vi "RT_test_ADC.vi"() -> ()   [LabVIEW 2018]
uses:
  <vilib>/Platform/TimedLoop/XDataNode/timing_clust.ctl
  <vilib>/Platform/TimedLoop/XDataNode/nitl_modes.ctl
  <vilib>/Platform/TimedLoop/XDataNode/wakeup.ctl
  Type Defs/BL Measurement States.ctl
  <vilib>/FPGAPlugInAG/myRIO-1900/niLvFpga_Open_myRIO-1900.vi
  <vilib>/rvi/interface/common/dynamic/niFpgaDynamicAddResources.vi
  <vilib>/Utility/error.llb/Error Cluster From Error Code.vi
  <vilib>/rvi/errors/niLvFpgaAdjustHostInterfaceError.vi
  <vilib>/rvi/interface/nirviOpenFPGA/nirviOpenFPGA.xnode
  UNCC Watt balance Oct19/FPGA Bitfiles/UNCCWattbalanceO_FPGATarget_fpganestedFORW&R_sb-Oe1PDHtY.lvbitx
  <vilib>/Platform/TimedLoop/XDataNode/XDataNode.xnode
  <vilib>/rvi/interface/nirviReadWriteControl/nirviReadWriteControl.xnode
  <vilib>/Platform/TimedLoop/XDataNode/XDNodeRunTimeDep.lvlib
  NiFpgaLv.dll
  <vilib>/rvi/interface/Simulation/niFpgaSimulationCallBeginRW.vi
panel:
  out "number of cycles":dbl
  out "Time period":dbl
  in  "no. datapoints":u16=1
  in  "gain":dbl=5.7903
  out "Velocity (m/s) 2":dbl=0.0007038140090386572
  out "displacement amplitude":dbl=0.0001120154785558262 format="%.6f"
  out "d input to Fourier":dbl[](graph)
  in  "Measure 2":bool
  out "Waveform Chart - Dark 2":dbl(graph)=-1.5424874498374959 caption="Waveform Chart - dark"
  out "Waveform Chart - Dark":dbl(graph)=0.00010993789767612186 caption="Waveform Chart - dark"
  out "Late? [i-1]":bool
  in  "delay (us)":u32=250
  in  "offset (mV)":dbl
  in  "amplitude (V)":dbl=0.8
  in  "frequency (Hz)":dbl=25.0
  in  "Stop Button":bool
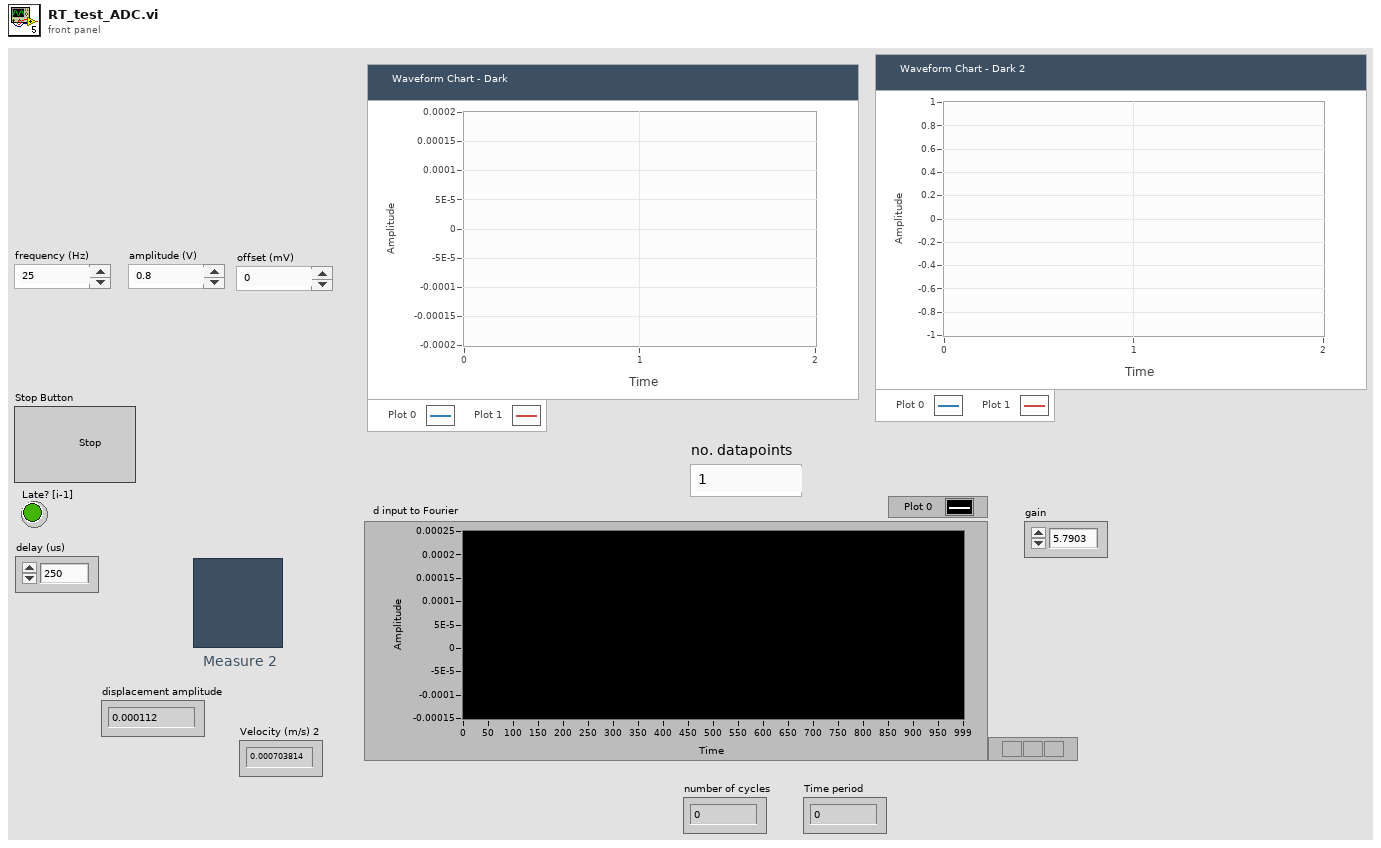
[diagram p1: front panel]
types:
  T1 = typedef "XDNodeRunTimeDep.lvlib/timing_clust.ctl" = cluster{"Expected End [f-1]":u64, "Actual End [f-1]":u64, "Finished Late? [f-1]":bool, "Expected End [i-1]":u64, "Actual End [i-1]":u64, "Finished Late? [i-1]":bool, "Expected Start [i]":u64, "Actual Start [i]":u64, "Expected Start [f]":u64, "Actual Start [f]":u64, "Source Name":string, "Structure Name":string, "Period":i64, "Deadline":i64, "Offset":i64, "Start":i64, "Priority":i32, "Timeout":i32, "Mode":T2, "Wakeup Reason":T3, "Error":errorcluster, "Source Type":string, "Secondary Source Type":string, "Global End Time":u64, "Global Start Time":u64, "Frame Duration":u64, "Iteration Duration":u64, "Assigned CPU":i32, "I/O Scan Engine Mode":u32}
  T2 = typedef "XDNodeRunTimeDep.lvlib/nitl_modes.ctl" = enum32{"No Change", "Process missed periods, maintain original phase", "Discard missed periods, maintain original phase", "Process missed periods, ignore original phase", "Discard missed periods, ignore original phase"}
  T3 = typedef "XDNodeRunTimeDep.lvlib/wakeup.ctl" = enum32{"Normal", "Aborted", "Asynchronous wakeup", "Timing source error", "Timed loop error", "Timeout"}
  T4 = typedef "BL Measurement States.ctl" = enum16{"idle", "initialize", "collect data", "prepare data", "fit sine", "calculate BL", "exit meas"}
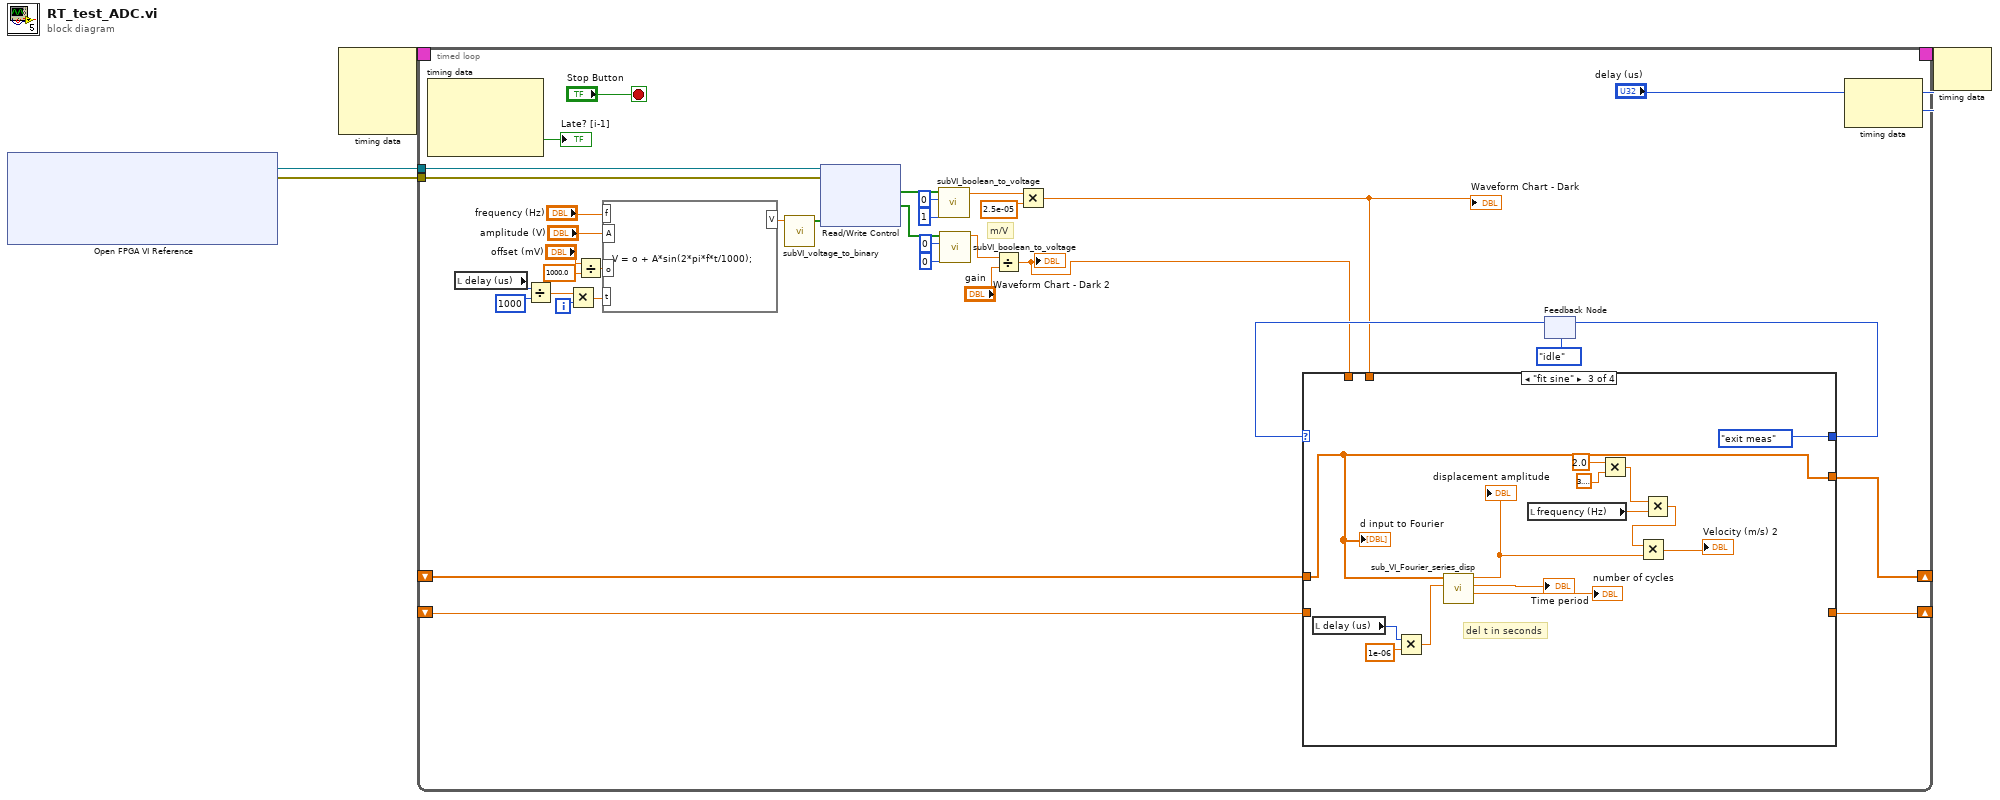
[diagram p0: block diagram]
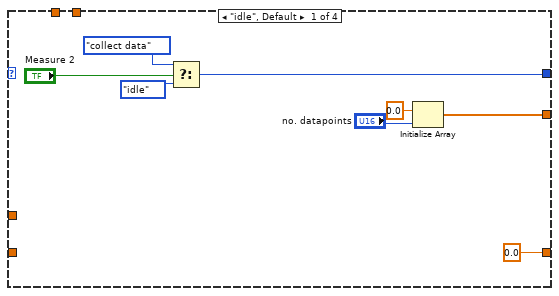
[diagram p2: hidden frame]
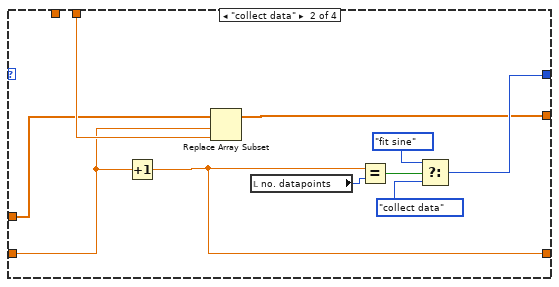
[diagram p3: hidden frame]
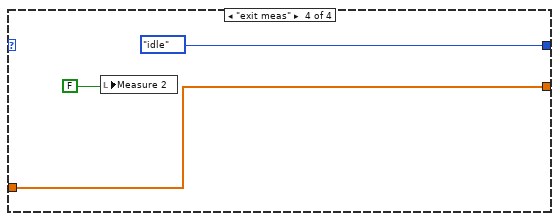
[diagram p4: hidden frame]
diagram:
  n1 = xnode "Open FPGA VI Reference"() -> ("FPGA VI Reference Out"=w4:refnum<k20>, "error out"=w3:errorcluster)  [unwired: 2 in]
  n2 = node-c288() -> (w2:T1)  [unwired: 4 in]
  n3 = timed-loop {
    tunnel: w4 -> [w40]
    tunnel: w3 -> [w39]
    timing: w2 -> [_]
    timing-out: [_] -> w1
    shift-right: [w14] -> _
    shift-left: _ -> [w13]
    shift-right: [w6] -> _
    shift-left: _ -> [w5]
    i -> [w19]
    stop <- "Stop Button" stop-if-true
    # "m/V"
    n4 = node-c288() -> (→"Late? [i-1]":bool)  [unwired: 1 in, 3 out]
    n5 = local read "delay (us)"() -> (w22:u32)
    n6 = Divide(x=w22, y=1000) -> (x/y=w20:dbl)
    n7 = Multiply(x=w20, y=w19) -> (x*y=w18:dbl)
    n8 = Divide(x="offset (mV)", y=1000.0) -> (x/y=w28:dbl)
    n9 = formula code="V = o + A*sin(2*pi*f*t/1000);"("f"="frequency (Hz)", "A"="amplitude (V)", "t"=w18, "o"=w28) -> ("V"=w27:dbl)
    n10 = call "subVI_voltage_to_binary.vi"("voltage"=w27) -> ("binary"=w26:bool[])  [unwired: 10 in]
    n11 = xnode "Read/Write Control"("FPGA VI Reference In"=w40, "error in"=w39, "DAC 1 write"=w26) -> ("ADC  1 R"=w7:bool[], "ADC 2 R"=w34:bool[])  [unwired: 2 out]
    n12 = call "subVI_boolean_to_voltage.vi"("Gain"=i16 1, "UNI"=i16 0, "ADC read"=w7) -> ("V"=w23:dbl)  [unwired: 8 in]
    n13 = call "subVI_boolean_to_voltage.vi"("Gain"=i16 0, "UNI"=i16 0, "ADC read"=w34) -> ("V"=w16:dbl)  [unwired: 8 in]
    n14 = Divide(x=w16, y="gain") -> (x/y=w8:dbl)
    "Waveform Chart - Dark 2" <- w8
    n15 = Multiply(x=w23, y=2.5e-05) -> (x*y=w10:dbl)
    "Waveform Chart - Dark" <- w10
    n16 = feedback #1(BL_Measurement_States."idle" ("BL meas states")) -> (w11:T4)
    n17 = case shown="\"fit sine\"" w11 {
      tunnel: [w46 w55 BL_Measurement_States."exit meas" ("BL meas states") BL_Measurement_States."idle" ("BL meas states")] -> w12
      tunnel: w10 -> [_ w53 _ _]
      tunnel: [w41 w54 w62 w73] -> w14
      tunnel: w13 -> [_ w52 w62 w73]
      tunnel: w8 -> [_ _ _ _]
      tunnel: [0.0 w51 _ _] -> w6
      tunnel: w5 -> [_ w50 _ _]
      frame "idle", Default {
        n18 = Select(t=BL_Measurement_States."collect data" ("BL meas states"), s="Measure 2", f=BL_Measurement_States."idle" ("BL meas states 2")) -> (s? t:f=w46:T4)
        n19 = Initialize Array(0.0 ("element"), "no. datapoints") -> (w41:dbl[])
      }
      frame "collect data" {
        n20 = Increment(x=w50) -> (x+1=w51:dbl)
        n21 = Replace Array Subset(array=w52, new element=w53, index=w50) -> (w54:dbl[])
        n22 = local read "no. datapoints"() -> (w49:u16)
        n23 = Equal?(x=w51, y=w49) -> (x = y?=w56:bool)
        n24 = Select(t=BL_Measurement_States."fit sine" ("BL meas states"), s=w56, f=BL_Measurement_States."collect data" ("BL meas states 2")) -> (s? t:f=w55:T4)
      }
      frame "fit sine" {
        # "del t in seconds"
        n25 = local read "delay (us)"() -> (w61:u32)
        n26 = Multiply(x=w61, y=1e-06) -> (x*y=w63:dbl)
        n27 = call "sub_VI_Fourier_series_disp.vi"("del t"=w63, "x,i"=w62) -> ("number of cycles"=→"number of cycles":dbl, "Time period"=→"Time period":dbl, "computed amplitude"=w67:dbl)  [unwired: 7 in]
        "displacement amplitude" <- w67
        n28 = local read "frequency (Hz)"() -> (w64:dbl)
        n29 = Multiply(x=2.0, y=3.141592653589793) -> (x*y=w70:dbl)
        n30 = Multiply(x=w70, y=w64) -> (x*y=w69:dbl)
        n31 = Multiply(x=w69, y=w67) -> (x*y=→"Velocity (m/s) 2":dbl)
        "d input to Fourier" <- w62
      }
      frame "exit meas" {
        n32 = local write "Measure 2"(FALSE) -> ()
      }
    }
    n33 = feedback-in #1(w12) -> ()
    n34 = node-c288("delay (us)") -> ()  [unwired: 1 in, 1 out]
  }
  n35 = node-c288(w1) -> ()  [unwired: 1 out]
